vi "PwF_ToF_HeartbeatRead.vi"() -> (0 "Firmware Rev":u16, 1 "Manuf PN":u16, 2 "Device ID":u8, 3 "Hardware SN":u32)   [LabVIEW 2018]
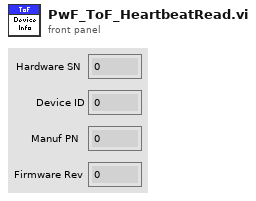
[diagram p1: front panel]
types:
  T1 = cluster{"Data[0]":u8, "Data[1]":u8, "Data[2]":u8, "Data[3]":u8, "Data[4]":u8, "Data[5]":u8, "Data[6]":u8, "Data[7]":u8, "Data[8]":u8}
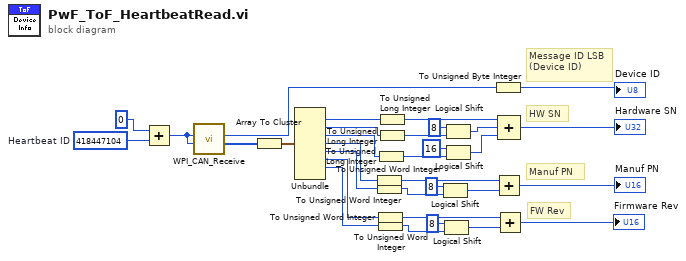
[diagram p0: block diagram]
diagram:
  w32 = u32 418447104  # Heartbeat ID
  # "Manuf PN"
  # "FW Rev"
  # "Message ID LSB\n(Device ID)"
  # "HW SN"
  n1 = Add(x=u32 0, y=w32) -> (x+y=w31:u32)
  n2 = call <vilib>:"WPI_CAN_Receive.vi"("Message ID Mask"=w31, "Message ID"=w31) -> ("Data"=w18:u8[], "Message ID Out"=w5:u32)  [unwired: 7 in, 1 out]
  n3 = Array To Cluster(array=w18) -> (cluster=w23:T1)
  n4 = Unbundle(w23) -> ("Data[1]"=w17:u8, "Data[2]"=w16:u8, "Data[3]"=w15:u8, "Data[4]"=w10:u8, "Data[5]"=w9:u8, "Data[6]"=w8:u8, "Data[7]"=w7:u8)  [unwired: 2 out]
  n5 = To Unsigned Word Integer(number=w10) -> (unsigned 16bit integer=w11:u16)
  n6 = To Unsigned Word Integer(number=w9) -> (unsigned 16bit integer=w12:u16)
  n7 = To Unsigned Word Integer(number=w8) -> (unsigned 16bit integer=w22:u16)
  n8 = To Unsigned Word Integer(number=w7) -> (unsigned 16bit integer=w24:u16)
  n9 = To Unsigned Long Integer(number=w15) -> (unsigned 32bit integer=w21:u32)
  n10 = To Unsigned Long Integer(number=w17) -> (unsigned 32bit integer=w19:u32)
  n11 = To Unsigned Long Integer(number=w16) -> (unsigned 32bit integer=w20:u32)
  n12 = Logical Shift(y=i16 8, x=w12) -> (x << y=w13:u16)
  n13 = Logical Shift(y=i16 8, x=w24) -> (x << y=w25:u16)
  n14 = Logical Shift(y=i16 8, x=w20) -> (x << y=w27:u32)
  n15 = Logical Shift(y=i16 16, x=w21) -> (x << y=w26:u32)
  n16 = To Unsigned Byte Integer(number=w5) -> (unsigned 8bit integer=→"Device ID":u8)
  n17 = Add(x=w11, y=w13) -> (x+y=→"Manuf PN":u16)
  n18 = Add(x=w22, y=w25) -> (x+y=→"Firmware Rev":u16)
  n19 = Compound Arithmetic op=ADD(w19, w27, w26) -> (→"Hardware SN":u32)
